vi "example_GProgramDownloadFile.vi"() -> ()   [LabVIEW 2020]
uses:
  <vilib>/Galil/resources/gclib32/gclib32.lvlib
  <vilib>/Galil/resources/gclibo32/gclibo32.lvlib
panel:
  in  "File Location":string="C:\\Program Files (x86)\\Galil\\gclib\\examples\\labview\\dmc_download.dmc"
  out "Error Out":errorcluster
  in  "IP Address":string="192.168.1.77"
  out "Response":string
  in  "Command":string="LS"
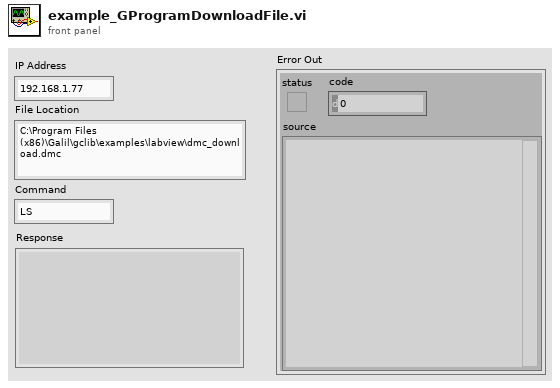
[diagram p1: front panel]
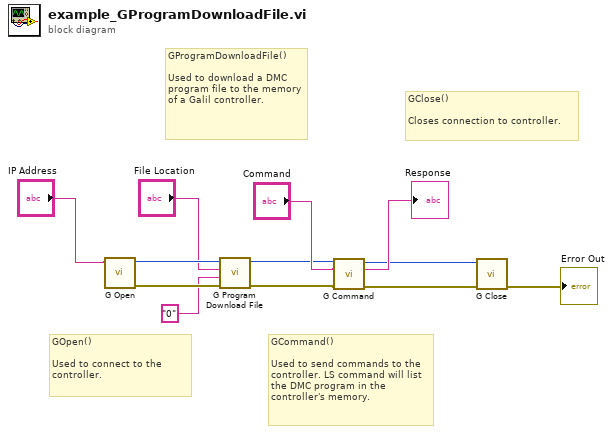
[diagram p0: block diagram]
diagram:
  # "GClose()\n\nCloses connection to controller."
  # "GCommand()\n\nUsed to send commands to the controller. LS command will list the DMC program in the controller's memory."
  # "GProgramDownloadFile()\n\nUsed to download a DMC  program file to the memory of a Galil controller."
  # "GOpen()\n\nUsed to connect to the controller."
  n1 = call <vilib>:"G Open.vi"("address"="IP Address") -> ("error out"=w4:errorcluster, "g out"=w6:u32)  [unwired: 8 in]
  n2 = call <vilib>:"G Program Download File.vi"("error in (no error)"=w4, "preprocessor"="0", "file_path"="File Location", "g"=w6) -> ("error out"=w3:errorcluster, "g out"=w2:u32)  [unwired: 6 in]
  n3 = call <vilib>:"G Command.vi"("g"=w2, "command"="Command", "error in (no error)"=w3) -> ("g out"=w8:u32, "buffer out"=→"Response":string, "error out"=w7:errorcluster)  [unwired: 10 in]
  n4 = call <vilib>:"G Close.vi"("error in (no error)"=w7, "g"=w8) -> ("error out"=→"Error Out":errorcluster)  [unwired: 9 in]
